vi "DBedit_init.vi"(7 "Pane":refnum<vi>, 8 "error in (no error)":errorcluster, 11 "DB-editor in":refnum<class "DB-editor.lvclass">) -> (0 "error out":errorcluster, 3 "DB-editor out":refnum<class "DB-editor.lvclass">)   [LabVIEW 2020, in "Sgraph_lib_V1.lvlib" / "DB-editor.lvclass"]
doc: "Andre Koelewijn, 18 aug 2021\n\nInitialization of the database editor application"
uses:
  DB-editor.lvclass
  <vilib>/Utility/miscctls.llb/LVPointTypeDef.ctl
  DB-editor.lvclass/DB-editor.ctl
  Gview/controls/Typedef_Gserver-Replies.ctl
  Gview/controls/Typedef_ServerActions.ctl
  Gserver/controls/Typedef_QueryType.ctl
  Gview/Gviewer.lvclass
  Gserver/Gserver.lvclass
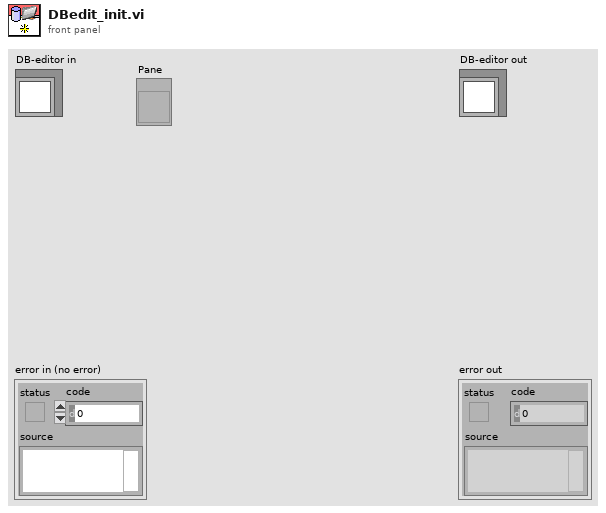
[diagram p1: front panel]
types:
  T1 = typedef "LVPointTypeDef.ctl" = cluster{"Horizontal":i16, "Vertical":i16}
  T2 = typedef "Typedef_Gserver-Replies.ctl" = cluster{"ServerActions":T3, "data":variant, "Source":string, "Time Stamp":timestamp}
  T3 = typedef "Sgraph_lib_V1.lvlib/Gviewer.lvclass/Typedef_ServerActions.ctl" = enum16{"GraphUpdate", "SendAllTags", "SendIniPath", "SetGeneralOptions", "EditTagsOpen", "EditTagsPresetSave", "EditTagsPresetLoad", "EditTagsClose", "NewTagSelection", "AutoScale", "DBeditStatus", "DBsaveConfirm", "GetXconstraints", "ExitGraph"}
  T4 = typedef "Sgraph_lib_V1.lvlib/Gserver.lvclass/Typedef_QueryType.ctl" = enum16{"Subscribe", "SubscribeNetw", "DataRequest", "RequestAllTags", "RequestIniPath", "FAMMstarted", "SetClientOptions", "GviewerUpdate", "OpenNewGraph", "CloseClient", "CloseAllClients", "Close Gserver", "OpenMemoryMap", "MeMapDataRequest", "MeMapDataResponse", "OpenDBeditor", "CheckDBeditorRunning", "StoppedDBeditor", "SaveDB_TAGpropRecord", "ConfirmDB_TAGpropSave", "GetXconstraints", "OpenNewNetworkGraph"}
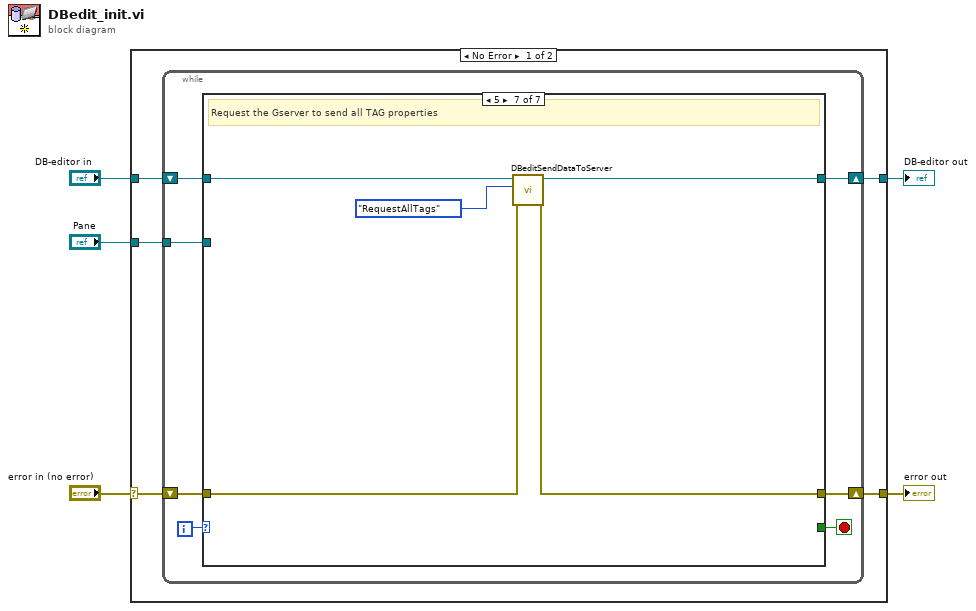
[diagram p0: block diagram]
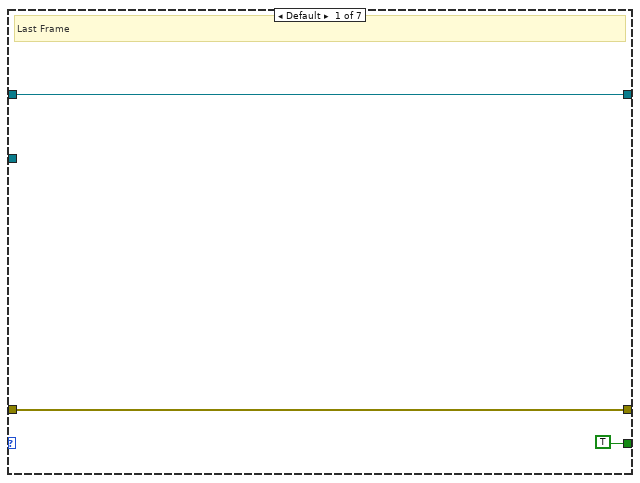
[diagram p2: hidden frame]
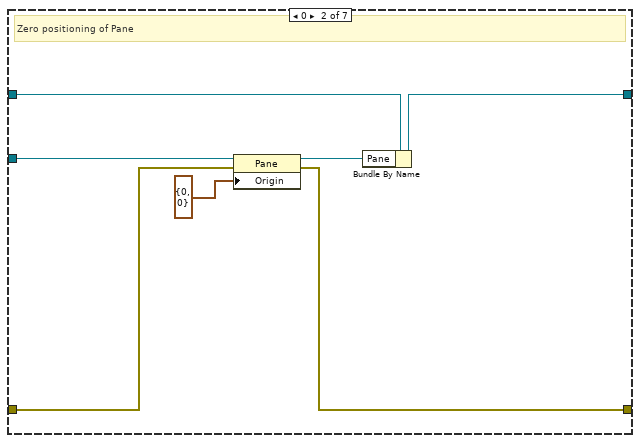
[diagram p3: hidden frame]
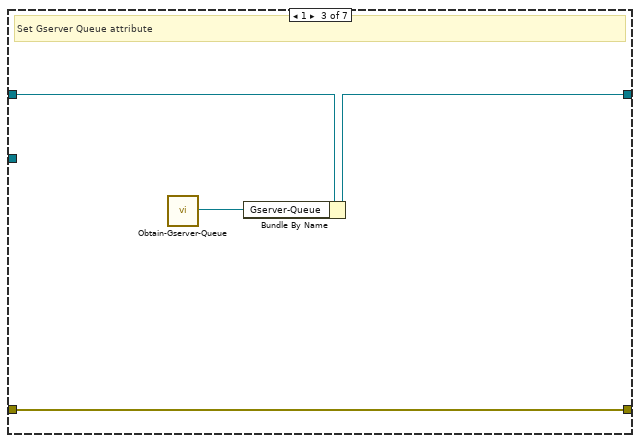
[diagram p4: hidden frame]
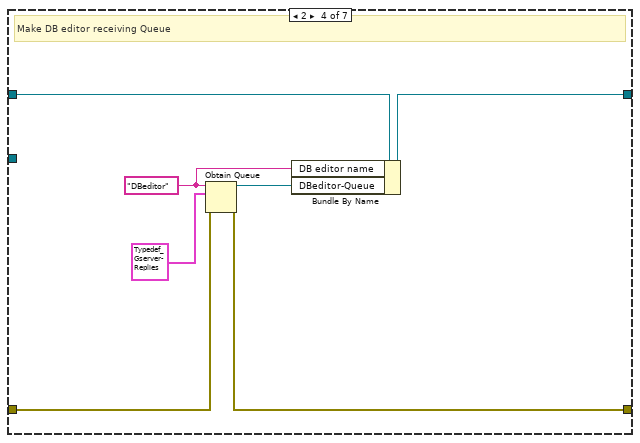
[diagram p5: hidden frame]
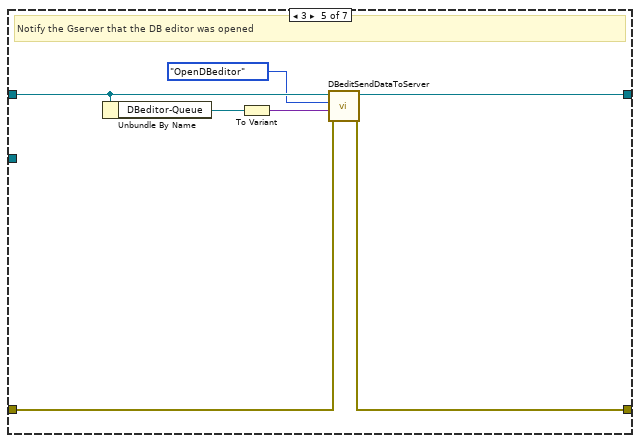
[diagram p6: hidden frame]
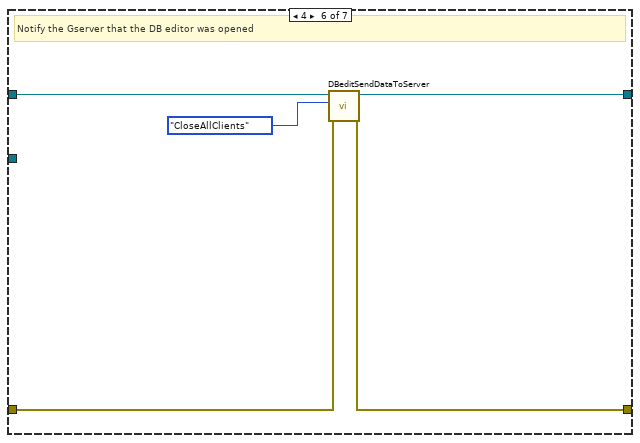
[diagram p7: hidden frame]
diagram:
  n1 = case shown="No Error" "error in (no error)" {
    selector: "error in (no error)" -> [w9 w57]
    tunnel: [w7 w57] -> w4
    tunnel: [w8 w56] -> w2
    tunnel: "DB-editor in" -> [w10 w56]
    tunnel: "Pane" -> [w6 _]
    frame No Error {
      n2 = while {
        shift-right: [w13] -> w7
        shift-left: w9 -> [w16]
        shift-right: [w14] -> w8
        shift-left: w10 -> [w15]
        tunnel: w6 -> [w11]
        i -> [w17]
        stop <- w12 stop-if-true
        n3 = case shown="5" w17 {
          tunnel: w16 -> [w20 w21 w29 w37 w44 w49 w54]
          tunnel: w15 -> [w18 w26 w31 w35 w42 w47 w52]
          tunnel: [w18 w27 w30 w33 w45 w50 w55] -> w14
          tunnel: [w20 w22 w29 w36 w43 w48 w53] -> w13
          tunnel: [TRUE _ _ _ _ _ _] -> w12
          tunnel: w11 -> [_ w23 _ _ _ _ _]
          frame Default {
            # "Last Frame"
          }
          frame 0 {
            # "Zero positioning of Pane"
            n4 = property class="Pane"(reference=w23, error in=w21, "Origin"=T1 {"Horizontal"=0, "Vertical"=0}) -> (reference out=w24:refnum<vi>, error out=w22:errorcluster)
            n5 = Bundle By Name(cluster=w26, "Pane"=w24) -> (w27:refnum<class "DB-editor.lvclass">)
          }
          frame 1 {
            # "Set Gserver Queue attribute"
            n6 = call "Obtain-Gserver-Queue.vi"() -> ("Gserver Queue"=w28:refnum<queue>)  [unwired: 7 in]
            n7 = Bundle By Name(cluster=w31, "Gserver-Queue"=w28) -> (w30:refnum<class "DB-editor.lvclass">)
          }
          frame 2 {
            w32 = "DBeditor" ("name (unnamed)")
            # "Make DB editor receiving Queue"
            n8 = Obtain Queue(name (unnamed)=w32, element data type=T2 {"ServerActions"=enum."GraphUpdate", "data"=variant, "Source"="", "Time Stamp"=timestamp(0 s since 1904-01-01)} ("Query"), error in (no error)=w37) -> (queue out=w34:refnum<queue>, error out=w36:errorcluster)  [unwired: 2 in, 1 out]
            n9 = Bundle By Name(cluster=w35, "DB editor name"=w32, "DBeditor-Queue"=w34) -> (w33:refnum<class "DB-editor.lvclass">)
          }
          frame 3 {
            # "Notify the Gserver that the DB editor was opened"
            n10 = Unbundle By Name(w42) -> ("DBeditor-Queue"=w41:refnum<queue>)
            n11 = To Variant(anything=w41) -> (Variant=w40:variant)
            n12 = call "DBeditSendDataToServer.vi"("error in (no error)"=w44, "data"=w40, "Query_type"=Typedef_QueryType."OpenDBeditor", "Gviewer in"=w42) -> ("error out"=w43:errorcluster, "Gviewer out"=w45:refnum<class "DB-editor.lvclass">)  [unwired: 6 in]
          }
          frame 4 {
            # "Notify the Gserver that the DB editor was opened"
            n13 = call "DBeditSendDataToServer.vi"("error in (no error)"=w49, "Query_type"=Typedef_QueryType."CloseAllClients", "Gviewer in"=w47) -> ("error out"=w48:errorcluster, "Gviewer out"=w50:refnum<class "DB-editor.lvclass">)  [unwired: 7 in]
          }
          frame 5 {
            # "Request the Gserver to send all TAG properties"
            n14 = call "DBeditSendDataToServer.vi"("error in (no error)"=w54, "Query_type"=Typedef_QueryType."RequestAllTags", "Gviewer in"=w52) -> ("error out"=w53:errorcluster, "Gviewer out"=w55:refnum<class "DB-editor.lvclass">)  [unwired: 7 in]
          }
        }
      }
    }
    frame Error {
    }
  }
  "error out" <- w4
  "DB-editor out" <- w2
